vi "glueAlignPinInsert_stereo.vi"() -> ()   [LabVIEW 2015]
uses:
  GlobalPath.vi
  GlobalData.vi
  GlobalVi.vi
panel:
  in  "ptfe 42":bool caption="Manually push down the two pins of the vertical positioning tool to insert them in the holes of the plates"
  in  "ptfe 41":bool caption="Manually push down the two pins of the vertical positioning tool to insert them in the holes of the plates"
  out "PanelName":string
  in  "ptfe 33":bool caption="Remove the electroerosion pin"
  in  "ptfe 39":bool caption="Insert the electroerosition pin in the slotted insert"
  in  "ptfe 31":bool caption="Check the planarity of the tool with the gauge machine"
  in  "ptfe 30":bool caption="Tighten the three screws to block the vertical positioning tool in place"
  in  "ptfe 29":bool caption="Check the planarity of the tool with the gauge machine"
  in  "ptfe 28":bool caption="Tighten the three screws to block the vertical positioning tool in place"
  in  "ptfe 27":bool caption="Position the alignment pin in the panel hole"
  in  "ptfe 26":bool caption="Position the panel on the table"
  in  "ptfe 25":bool caption="Move the panel away from the table"
  in  "ptfe 24":bool caption="Lift the panel from the table"
  in  "ptfe 23":bool caption="Switch on the vacuum on the machine"
  in  "ptfe 22":bool caption="Lower the machine on the panel"
  in  "ptfe 21":bool caption="Move the rotating machine on top of the panel"
  in  "Done ?":bool
  in  "ptfe 20":bool caption="Wait 24h for the glue to cure"
  in  "ptfe 19":bool caption="Position the reinforcing washers on the emerging part of the alignment pins and insert"
  in  "ptfe 18":bool caption="Deposit the glue on the emerging part of the alignment pins and insert using a thin needle"
  in  "ptfe 17":bool caption="Rotate the panel so that it's back side is up"
  in  "ptfe 16":bool caption="Switch off the vacuum"
  in  "ptfe 15":bool caption="Remove the three vertical positioning tools, blocking plates and positioning pins"
  in  "ptfe 14":bool caption="Wait 24h for the glue to cure"
  in  "ptfe 13":bool caption="Place and screw the blocking plate to the vertical positioning tool to keep the pin orthogonality during the curing of the glue"
  in  "ptfe 12":bool caption="Position the vertical positioning tool on the reference plate with its positioning pins"
  in  "ptfe 11":bool caption="Deposit the glue on the stainless steel slotted insert grooves"
  in  "ptfe 9":bool caption="Position the insert in the dedicated hole on the panel"
  in  "ptfe 8":bool caption="Repeat these steps in order to glue the second alignment pin on the other side of the panel"
  in  "ptfe 7":bool caption="Place and screw the blocking plate to the vertical positioning tool to keep the pin orthogonality during the curing of the glue"
  in  "ptfe 5":bool caption="Position the vertical positioning tool on the reference plate with its positioning pins"
  in  "ptfe 4":bool caption="Deposit the glue on the precise alignment pin grooves"
  in  "ptfe 2":bool caption="Check that the vacuum is on"
  # "Gluing of Alignment Pin/Insert"
  # "STEREO PANEL \nINSTRUCTIONS"
  # "GLUING OF THE TWO PINS"
  # "GLUING OF THE HARDENED STEEL INSERT"
  # "Add info on Enumeration"
  # "COMMON PROCEDURE"
  # "GLUE CURING OF THE TWO PINS AND INSERT"
  # "GLUING OF REINFORCING WASHER ON PANEL BACK SIDE"
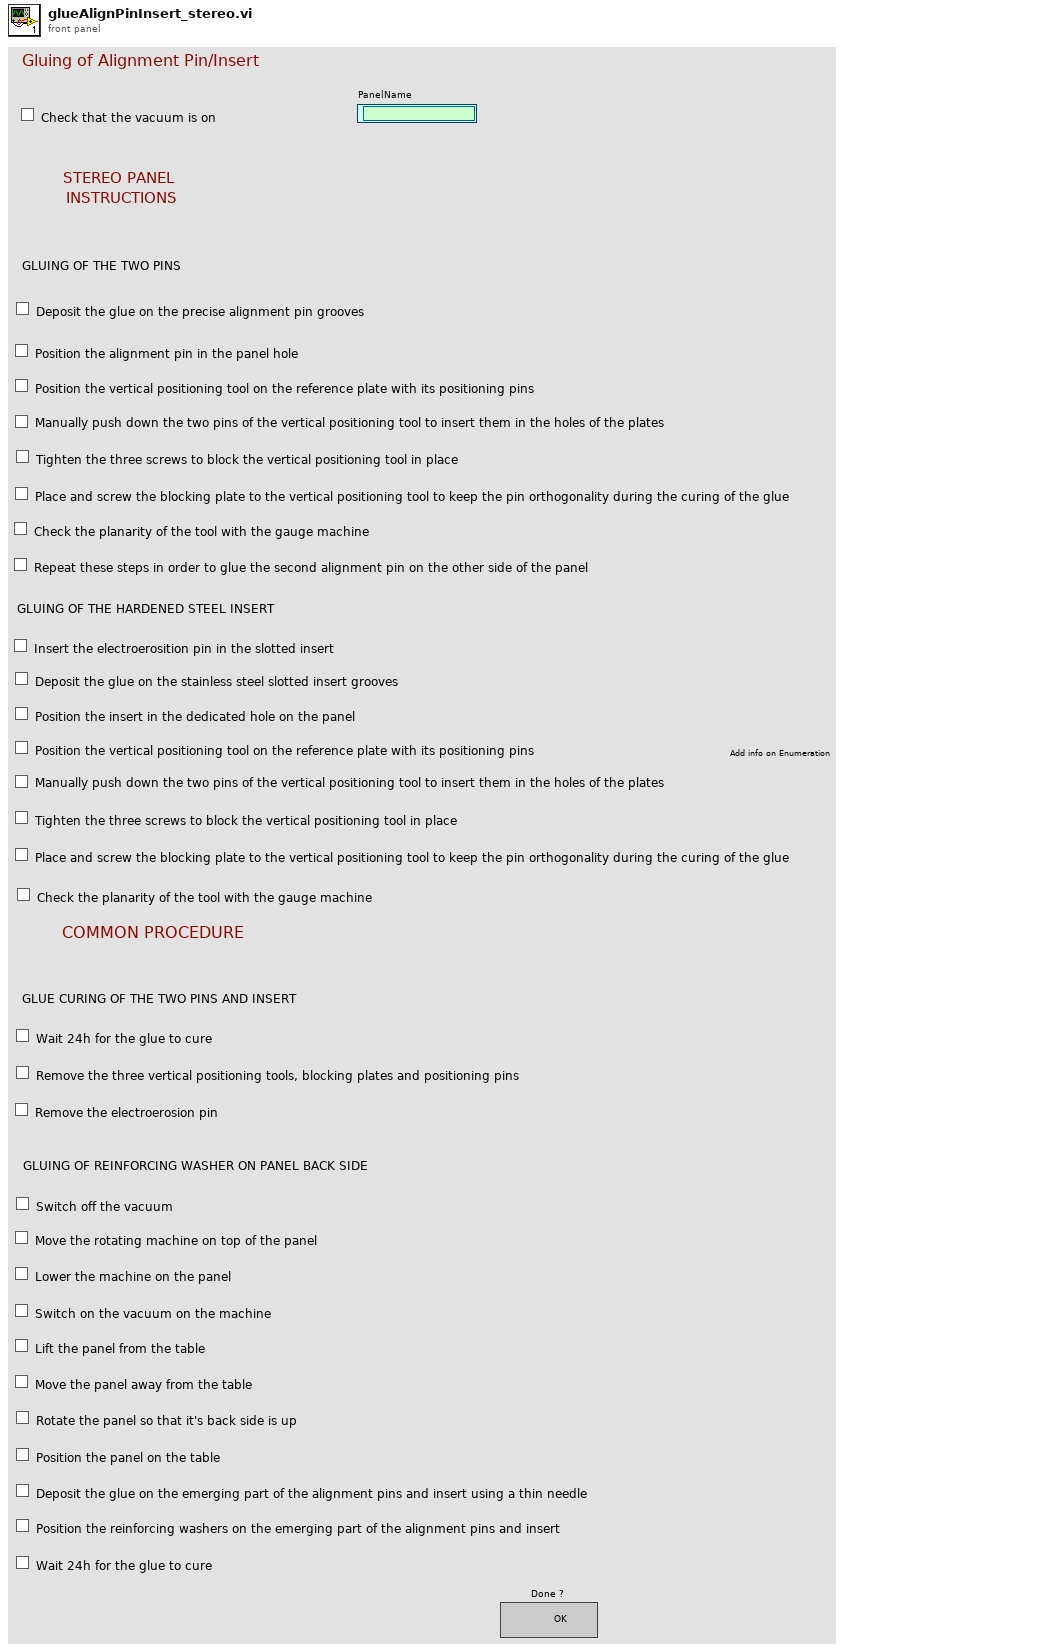
[diagram p1: front panel]
types:
  T1 = enum16{"open", "replace", "create", "open or create", "replace or create", "replace or create with confirmation"}
  T2 = enum32{"Bad", "Idle", "Run top level", "Running"}
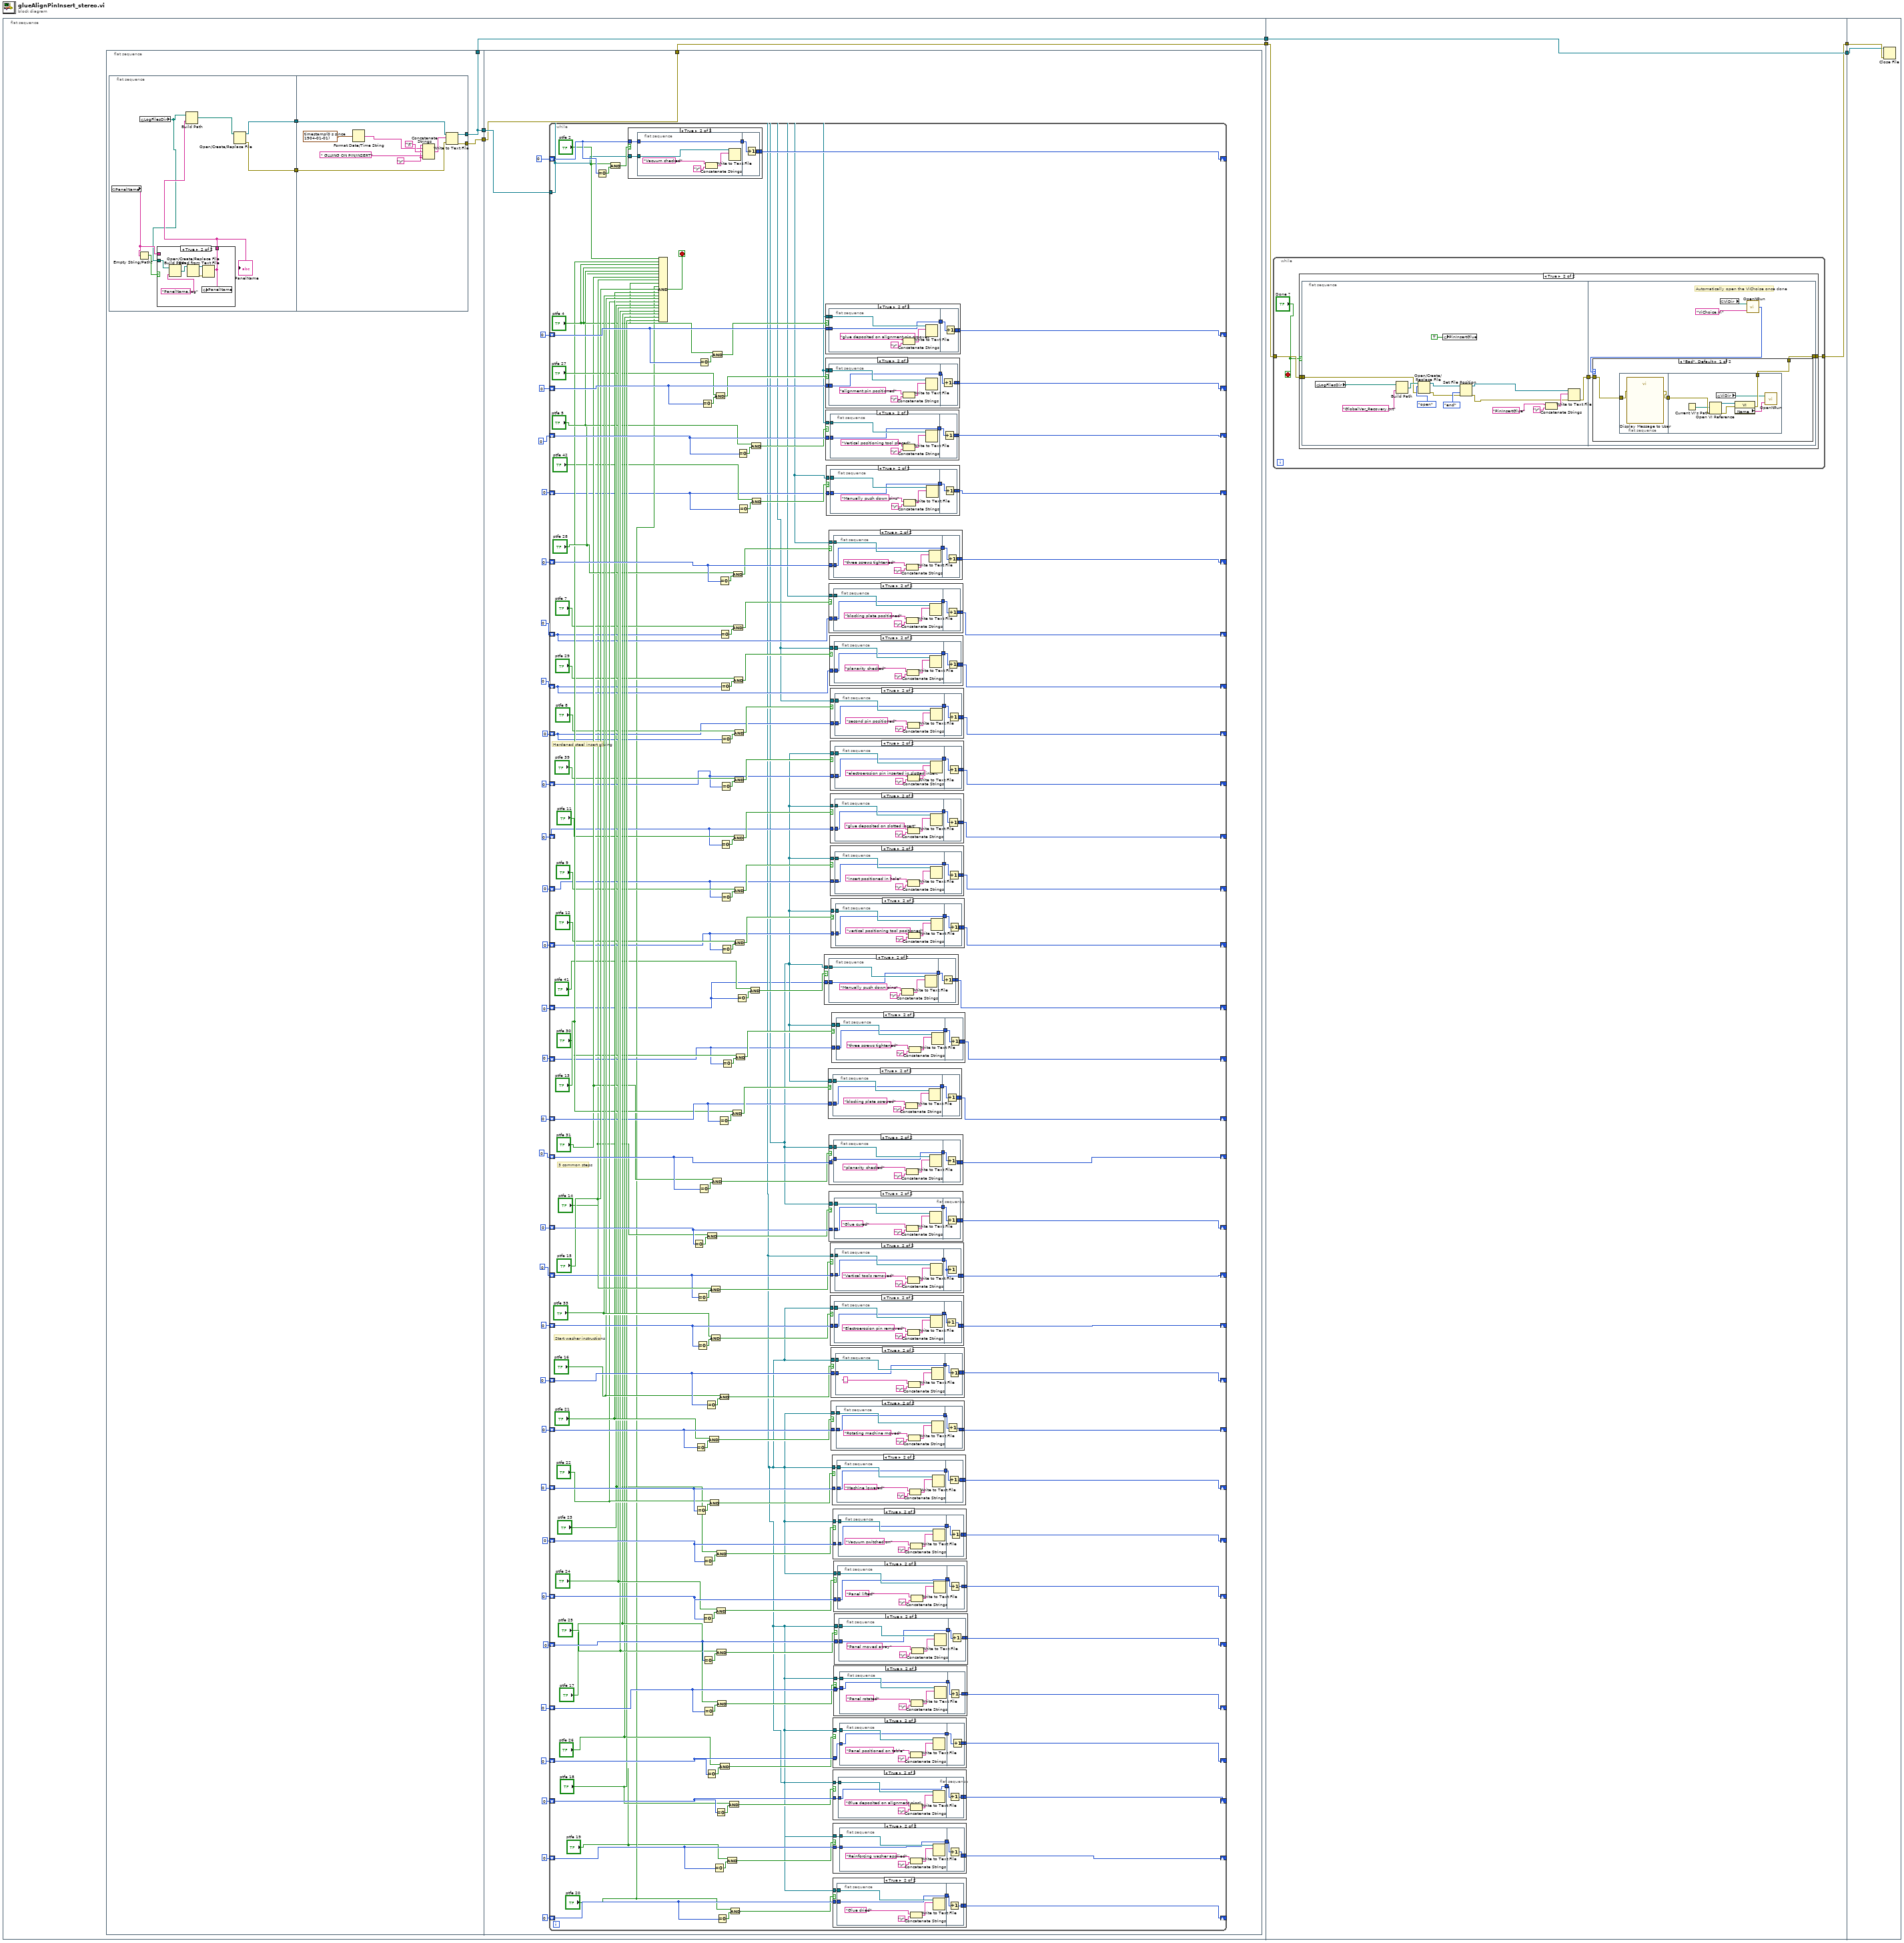
[diagram p0: block diagram]
diagram:
  n1 = flat-sequence {
    tunnel: [w5] -> w3
    tunnel: [w7] -> w2
    tunnel: [w598] -> w4
    tunnel: w3 -> [w599]
    tunnel: w2 -> [w600]
    tunnel: [w600] -> w1
    tunnel: w4 -> [w644]
    tunnel: w1 -> [w643]
    frame #0 {
      n2 = flat-sequence {
        tunnel: [w11] -> w8
        tunnel: [w11] -> w7
        tunnel: [w9] -> w6
        tunnel: w8 -> [w69]
        tunnel: w6 -> [w68]
        tunnel: [w68] -> w5
        frame #0 {
          n3 = flat-sequence {
            tunnel: [w18] -> w12
            tunnel: [w17] -> w10
            tunnel: w12 -> [w31]
            tunnel: [w30] -> w11
            tunnel: [w29] -> w9
            tunnel: w10 -> [w28]
            frame #0 {
              n4 = global read "GlobalData.vi" "PanelName"() -> (w16:string)
              n5 = Empty String/Path?(string/path=w16) -> (empty?=w15:bool)
              n6 = global read "GlobalPath.vi" "LogFilesDir"() -> (w13:path)
              n7 = case shown="True" w15 {
                tunnel: w13 -> [_ w26]
                tunnel: [w20 w21] -> w14
                tunnel: w16 -> [w20 _]
                frame False {
                }
                frame True {
                  n8 = Build Path(base path=w26, name or relative path="PanelName.log") -> (appended path=w25:path)
                  n9 = Open/Create/Replace File(file path (use dialog)=w25) -> (refnum out=w22:refnum<file>, error out=w23:errorcluster)  [unwired: 5 in, 1 out]
                  n10 = Read from Text File(file (use dialog)=w22, error in=w23) -> (text=w21:string)  [unwired: 2 in, 3 out]
                  n11 = global write "GlobalData.vi" "PanelName"(w21) -> ()
                }
              }
              "PanelName" <- w14
              n12 = Build Path(base path=w13, name or relative path=w14) -> (appended path=w19:path)
              n13 = Open/Create/Replace File(file path (use dialog)=w19) -> (refnum out=w18:refnum<file>, error out=w17:errorcluster)  [unwired: 5 in, 1 out]
            }
            frame #1 {
              w27 = "\r"
              n14 = Format Date/Time String(seconds (now)=timestamp(0 s since 1904-01-01)) -> (date/time string=w34:string)  [unwired: 2 in]
              n15 = Concatenate Strings(w27, w34, "\t", " GLUING ON PIN/INSERT", w27) -> (w32:string)
              n16 = Write to Text File(file (use dialog)=w31, text=w32, error in=w28) -> (refnum out=w30:refnum<file>, error out=w29:errorcluster)  [unwired: 1 in, 1 out]
            }
          }
        }
        frame #1 {
          n17 = while {
            tunnel: w69 -> [w73]
            shift-right: [w225] -> _
            shift-left: 0 -> [w204]
            shift-right: [w224] -> _
            shift-left: 0 -> [w196]
            shift-right: [w223] -> _
            shift-left: 0 -> [w195]
            shift-right: [w222] -> _
            shift-left: 0 -> [w194]
            shift-right: [w221] -> _
            shift-left: 0 -> [w190]
            shift-right: [w220] -> _
            shift-left: 0 -> [w188]
            shift-right: [w219] -> _
            shift-left: 0 -> [w183]
            shift-right: [w218] -> _
            shift-left: 0 -> [w180]
            shift-right: [w217] -> _
            shift-left: 0 -> [w178]
            shift-right: [w216] -> _
            shift-left: 0 -> [w167]
            shift-right: [w215] -> _
            shift-left: 0 -> [w166]
            shift-right: [w214] -> _
            shift-left: 0 -> [w165]
            shift-right: [w213] -> _
            shift-left: 0 -> [w164]
            shift-right: [w212] -> _
            shift-left: 0 -> [w163]
            shift-right: [w211] -> _
            shift-left: 0 -> [w162]
            shift-right: [w210] -> _
            shift-left: 0 -> [w161]
            shift-right: [w209] -> _
            shift-left: 0 -> [w160]
            shift-right: [w208] -> _
            shift-left: 0 -> [w159]
            shift-right: [w207] -> _
            shift-left: 0 -> [w139]
            shift-right: [w206] -> _
            shift-left: 0 -> [w138]
            shift-right: [w132] -> _
            shift-left: 0 -> [w133]
            shift-right: [w93] -> _
            shift-left: 0 -> [w101]
            shift-right: [w86] -> _
            shift-left: 0 -> [w100]
            shift-right: [w87] -> _
            shift-left: 0 -> [w99]
            shift-right: [w88] -> _
            shift-left: 0 -> [w98]
            shift-right: [w89] -> _
            shift-left: 0 -> [w97]
            shift-right: [w90] -> _
            shift-left: 0 -> [w96]
            shift-right: [w91] -> _
            shift-left: 0 -> [w95]
            shift-right: [w92] -> _
            shift-left: 0 -> [w94]
            shift-right: [w76] -> _
            shift-left: 0 -> [w77]
            shift-right: [w70] -> _
            shift-left: 0 -> [w71]
            stop <- w226 stop-if-true
            # "Hardened steel insert gluing"
            # "3 common steps"
            # "Start washer instructions"
            n18 = Equal To 0?(x=w204) -> (x = 0?=w205:bool)
            n19 = And(x="ptfe 2", y=w205) -> (x .and. y?=w202:bool)
            n20 = case shown="True" w202 {
              tunnel: w73 -> [_ w590]
              tunnel: w204 -> [w586 w589]
              tunnel: [w586 w587] -> w225
              frame False {
              }
              frame True {
                n21 = flat-sequence {
                  tunnel: w590 -> [w592]
                  tunnel: w589 -> [w591]
                  tunnel: [w591] -> w588
                  tunnel: w588 -> [w597]
                  tunnel: [w596] -> w587
                  frame #0 {
                    n22 = Concatenate Strings("Vacuum checked", "\r") -> (w595:string)
                    n23 = Write to Text File(file (use dialog)=w592, text=w595) -> ()  [unwired: 2 in, 3 out]
                  }
                  frame #1 {
                    n24 = Increment(x=w597) -> (x+1=w596:i32)
                  }
                }
              }
            }
            n25 = Compound Arithmetic op=AND("ptfe 2", "ptfe 13", "ptfe 4", "ptfe 4", "ptfe 5", "ptfe 28", "ptfe 31", "ptfe 14", "ptfe 19", "ptfe 20", "ptfe 15", "ptfe 21", "ptfe 33", "ptfe 16", "ptfe 22", "ptfe 23", "ptfe 24", "ptfe 25", "ptfe 17", "ptfe 26", "ptfe 18") -> (w226:bool)
            n26 = Equal To 0?(x=w183) -> (x = 0?=w186:bool)
            n27 = Equal To 0?(x=w166) -> (x = 0?=w175:bool)
            n28 = Equal To 0?(x=w165) -> (x = 0?=w174:bool)
            n29 = Equal To 0?(x=w180) -> (x = 0?=w185:bool)
            n30 = Equal To 0?(x=w178) -> (x = 0?=w184:bool)
            n31 = Equal To 0?(x=w188) -> (x = 0?=w197:bool)
            n32 = Equal To 0?(x=w196) -> (x = 0?=w201:bool)
            n33 = Equal To 0?(x=w195) -> (x = 0?=w200:bool)
            n34 = Equal To 0?(x=w163) -> (x = 0?=w172:bool)
            n35 = Equal To 0?(x=w164) -> (x = 0?=w173:bool)
            n36 = Equal To 0?(x=w162) -> (x = 0?=w171:bool)
            n37 = Equal To 0?(x=w161) -> (x = 0?=w170:bool)
            n38 = Equal To 0?(x=w167) -> (x = 0?=w176:bool)
            n39 = Equal To 0?(x=w160) -> (x = 0?=w169:bool)
            n40 = And(x="ptfe 14", y=w186) -> (x .and. y?=w182:bool)
            n41 = And(x="ptfe 21", y=w175) -> (x .and. y?=w154:bool)
            n42 = And(x="ptfe 22", y=w174) -> (x .and. y?=w152:bool)
            n43 = And(x="ptfe 15", y=w185) -> (x .and. y?=w179:bool)
            n44 = And(x="ptfe 33", y=w184) -> (x .and. y?=w177:bool)
            n45 = And(x="ptfe 31", y=w197) -> (x .and. y?=w187:bool)
            n46 = And(x="ptfe 4", y=w201) -> (x .and. y?=w193:bool)
            n47 = Equal To 0?(x=w139) -> (x = 0?=w141:bool)
            n48 = And(x="ptfe 27", y=w200) -> (x .and. y?=w192:bool)
            n49 = And(x="ptfe 24", y=w172) -> (x .and. y?=w150:bool)
            n50 = Equal To 0?(x=w159) -> (x = 0?=w168:bool)
            n51 = And(x="ptfe 23", y=w173) -> (x .and. y?=w85:bool)
            n52 = And(x="ptfe 25", y=w171) -> (x .and. y?=w148:bool)
            n53 = And(x="ptfe 17", y=w170) -> (x .and. y?=w146:bool)
            n54 = Equal To 0?(x=w138) -> (x = 0?=w140:bool)
            n55 = Equal To 0?(x=w133) -> (x = 0?=w135:bool)
            n56 = Equal To 0?(x=w190) -> (x = 0?=w198:bool)
            n57 = And(x="ptfe 16", y=w176) -> (x .and. y?=w156:bool)
            n58 = Equal To 0?(x=w100) -> (x = 0?=w125:bool)
            n59 = And(x="ptfe 26", y=w169) -> (x .and. y?=w144:bool)
            n60 = Equal To 0?(x=w99) -> (x = 0?=w123:bool)
            n61 = Equal To 0?(x=w96) -> (x = 0?=w117:bool)
            n62 = Equal To 0?(x=w98) -> (x = 0?=w121:bool)
            n63 = Equal To 0?(x=w97) -> (x = 0?=w119:bool)
            n64 = Equal To 0?(x=w95) -> (x = 0?=w115:bool)
            n65 = Equal To 0?(x=w94) -> (x = 0?=w113:bool)
            n66 = Equal To 0?(x=w101) -> (x = 0?=w111:bool)
            n67 = And(x="ptfe 19", y=w141) -> (x .and. y?=w137:bool)
            n68 = And(x="ptfe 18", y=w168) -> (x .and. y?=w142:bool)
            n69 = And(x="ptfe 20", y=w140) -> (x .and. y?=w136:bool)
            n70 = And(x="ptfe 13", y=w135) -> (x .and. y?=w134:bool)
            n71 = And(x="ptfe 28", y=w198) -> (x .and. y?=w189:bool)
            n72 = And(x="ptfe 7", y=w125) -> (x .and. y?=w124:bool)
            n73 = And(x="ptfe 29", y=w123) -> (x .and. y?=w122:bool)
            n74 = And(x="ptfe 11", y=w117) -> (x .and. y?=w116:bool)
            n75 = And(x="ptfe 8", y=w121) -> (x .and. y?=w120:bool)
            n76 = And(x="ptfe 39", y=w119) -> (x .and. y?=w118:bool)
            n77 = And(x="ptfe 9", y=w115) -> (x .and. y?=w114:bool)
            n78 = And(x="ptfe 12", y=w113) -> (x .and. y?=w112:bool)
            n79 = And(x="ptfe 30", y=w111) -> (x .and. y?=w110:bool)
            n80 = Equal To 0?(x=w71) -> (x = 0?=w75:bool)
            n81 = Equal To 0?(x=w194) -> (x = 0?=w199:bool)
            n82 = Equal To 0?(x=w77) -> (x = 0?=w80:bool)
            n83 = And(x="ptfe 41", y=w75) -> (x .and. y?=w74:bool)
            n84 = And(x="ptfe 5", y=w199) -> (x .and. y?=w191:bool)
            n85 = And(x="ptfe 42", y=w80) -> (x .and. y?=w79:bool)
            n86 = case shown="True" w74 {
              tunnel: w73 -> [_ w231]
              tunnel: w71 -> [w227 w229]
              tunnel: [w227 w228] -> w70
              frame False {
              }
              frame True {
                n87 = flat-sequence {
                  tunnel: w231 -> [w233]
                  tunnel: [w232] -> w230
                  tunnel: w229 -> [w232]
                  tunnel: w230 -> [w238]
                  tunnel: [w237] -> w228
                  frame #0 {
                    n88 = Concatenate Strings("Manually push down pins", "\r") -> (w236:string)
                    n89 = Write to Text File(file (use dialog)=w233, text=w236) -> ()  [unwired: 2 in, 3 out]
                  }
                  frame #1 {
                    n90 = Increment(x=w238) -> (x+1=w237:i32)
                  }
                }
              }
            }
            n91 = case shown="True" w192 {
              tunnel: w73 -> [_ w566]
              tunnel: w195 -> [w562 w564]
              tunnel: [w562 w563] -> w223
              frame False {
              }
              frame True {
                n92 = flat-sequence {
                  tunnel: w566 -> [w568]
                  tunnel: [w567] -> w565
                  tunnel: w564 -> [w567]
                  tunnel: w565 -> [w573]
                  tunnel: [w572] -> w563
                  frame #0 {
                    n93 = Concatenate Strings("alignment pin positioned", "\r") -> (w571:string)
                    n94 = Write to Text File(file (use dialog)=w568, text=w571) -> ()  [unwired: 2 in, 3 out]
                  }
                  frame #1 {
                    n95 = Increment(x=w573) -> (x+1=w572:i32)
                  }
                }
              }
            }
            n96 = case shown="True" w193 {
              tunnel: w73 -> [_ w578]
              tunnel: w196 -> [w574 w577]
              tunnel: [w574 w575] -> w224
              frame False {
              }
              frame True {
                n97 = flat-sequence {
                  tunnel: w578 -> [w580]
                  tunnel: w577 -> [w579]
                  tunnel: [w579] -> w576
                  tunnel: w576 -> [w585]
                  tunnel: [w584] -> w575
                  frame #0 {
                    n98 = Concatenate Strings("glue deposited on alignment pin grooves", "\r") -> (w583:string)
                    n99 = Write to Text File(file (use dialog)=w580, text=w583) -> ()  [unwired: 2 in, 3 out]
                  }
                  frame #1 {
                    n100 = Increment(x=w585) -> (x+1=w584:i32)
                  }
                }
              }
            }
            n101 = case shown="True" w191 {
              tunnel: w73 -> [_ w554]
              tunnel: w194 -> [w550 w552]
              tunnel: [w550 w551] -> w222
              frame False {
              }
              frame True {
                n102 = flat-sequence {
                  tunnel: w554 -> [w556]
                  tunnel: [w555] -> w553
                  tunnel: w552 -> [w555]
                  tunnel: w553 -> [w561]
                  tunnel: [w560] -> w551
                  frame #0 {
                    n103 = Concatenate Strings("Vertical positioning tool placed", "\r") -> (w559:string)
                    n104 = Write to Text File(file (use dialog)=w556, text=w559) -> ()  [unwired: 2 in, 3 out]
                  }
                  frame #1 {
                    n105 = Increment(x=w561) -> (x+1=w560:i32)
                  }
                }
              }
            }
            n106 = case shown="True" w79 {
              tunnel: w73 -> [_ w243]
              tunnel: w77 -> [w239 w241]
              tunnel: [w239 w240] -> w76
              frame False {
              }
              frame True {
                n107 = flat-sequence {
                  tunnel: w243 -> [w245]
                  tunnel: [w244] -> w242
                  tunnel: w241 -> [w244]
                  tunnel: w242 -> [w250]
                  tunnel: [w249] -> w240
                  frame #0 {
                    n108 = Concatenate Strings("Manually push down pins", "\r") -> (w248:string)
                    n109 = Write to Text File(file (use dialog)=w245, text=w248) -> ()  [unwired: 2 in, 3 out]
                  }
                  frame #1 {
                    n110 = Increment(x=w250) -> (x+1=w249:i32)
                  }
                }
              }
            }
            n111 = case shown="True" w134 {
              tunnel: w73 -> [_ w351]
              tunnel: w133 -> [w347 w349]
              tunnel: [w347 w348] -> w132
              frame False {
              }
              frame True {
                n112 = flat-sequence {
                  tunnel: w351 -> [w353]
                  tunnel: [w352] -> w350
                  tunnel: w349 -> [w352]
                  tunnel: w350 -> [w358]
                  tunnel: [w357] -> w348
                  frame #0 {
                    n113 = Concatenate Strings("blocking plate screwed", "\r") -> (w356:string)
                    n114 = Write to Text File(file (use dialog)=w353, text=w356) -> ()  [unwired: 2 in, 3 out]
                  }
                  frame #1 {
                    n115 = Increment(x=w358) -> (x+1=w357:i32)
                  }
                }
              }
            }
            n116 = case shown="True" w189 {
              tunnel: w73 -> [_ w530]
              tunnel: w190 -> [w526 w528]
              tunnel: [w526 w527] -> w221
              frame False {
              }
              frame True {
                n117 = flat-sequence {
                  tunnel: w530 -> [w532]
                  tunnel: [w531] -> w529
                  tunnel: w528 -> [w531]
                  tunnel: w529 -> [w537]
                  tunnel: [w536] -> w527
                  frame #0 {
                    n118 = Concatenate Strings("three screws tightened", "\r") -> (w535:string)
                    n119 = Write to Text File(file (use dialog)=w532, text=w535) -> ()  [unwired: 2 in, 3 out]
                  }
                  frame #1 {
                    n120 = Increment(x=w537) -> (x+1=w536:i32)
                  }
                }
              }
            }
            n121 = case shown="True" w124 {
              tunnel: w73 -> [_ w339]
              tunnel: w100 -> [w335 w337]
              tunnel: [w335 w336] -> w86
              frame False {
              }
              frame True {
                n122 = flat-sequence {
                  tunnel: w339 -> [w341]
                  tunnel: [w340] -> w338
                  tunnel: w337 -> [w340]
                  tunnel: w338 -> [w346]
                  tunnel: [w345] -> w336
                  frame #0 {
                    n123 = Concatenate Strings("blocking plate positioned", "\r") -> (w344:string)
                    n124 = Write to Text File(file (use dialog)=w341, text=w344) -> ()  [unwired: 2 in, 3 out]
                  }
                  frame #1 {
                    n125 = Increment(x=w346) -> (x+1=w345:i32)
                  }
                }
              }
            }
            n126 = case shown="True" w187 {
              tunnel: w73 -> [_ w542]
              tunnel: w188 -> [w538 w541]
              tunnel: [w538 w539] -> w220
              frame False {
              }
              frame True {
                n127 = flat-sequence {
                  tunnel: w542 -> [w544]
                  tunnel: w541 -> [w543]
                  tunnel: [w543] -> w540
                  tunnel: w540 -> [w549]
                  tunnel: [w548] -> w539
                  frame #0 {
                    n128 = Concatenate Strings("planarity checked", "\r") -> (w547:string)
                    n129 = Write to Text File(file (use dialog)=w544, text=w547) -> ()  [unwired: 2 in, 3 out]
                  }
                  frame #1 {
                    n130 = Increment(x=w549) -> (x+1=w548:i32)
                  }
                }
              }
            }
            n131 = case shown="True" w182 {
              tunnel: w73 -> [_ w518]
              tunnel: w183 -> [w514 w516]
              tunnel: [w514 w515] -> w219
              frame False {
              }
              frame True {
                n132 = flat-sequence {
                  tunnel: w518 -> [w520]
                  tunnel: [w519] -> w517
                  tunnel: w516 -> [w519]
                  tunnel: w517 -> [w525]
                  tunnel: [w524] -> w515
                  frame #0 {
                    n133 = Concatenate Strings("Glue cured", "\r") -> (w523:string)
                    n134 = Write to Text File(file (use dialog)=w520, text=w523) -> ()  [unwired: 2 in, 3 out]
                  }
                  frame #1 {
                    n135 = Increment(x=w525) -> (x+1=w524:i32)
                  }
                }
              }
            }
            n136 = case shown="True" w122 {
              tunnel: w73 -> [_ w327]
              tunnel: w99 -> [w323 w325]
              tunnel: [w323 w324] -> w87
              frame False {
              }
              frame True {
                n137 = flat-sequence {
                  tunnel: w327 -> [w329]
                  tunnel: [w328] -> w326
                  tunnel: w325 -> [w328]
                  tunnel: w326 -> [w334]
                  tunnel: [w333] -> w324
                  frame #0 {
                    n138 = Concatenate Strings("planarity checked", "\r") -> (w332:string)
                    n139 = Write to Text File(file (use dialog)=w329, text=w332) -> ()  [unwired: 2 in, 3 out]
                  }
                  frame #1 {
                    n140 = Increment(x=w334) -> (x+1=w333:i32)
                  }
                }
              }
            }
            n141 = case shown="True" w116 {
              tunnel: w73 -> [_ w291]
              tunnel: w96 -> [w287 w289]
              tunnel: [w287 w288] -> w90
              frame False {
              }
              frame True {
                n142 = flat-sequence {
                  tunnel: w291 -> [w293]
                  tunnel: [w292] -> w290
                  tunnel: w289 -> [w292]
                  tunnel: w290 -> [w298]
                  tunnel: [w297] -> w288
                  frame #0 {
                    n143 = Concatenate Strings("glue deposited on slotted insert", "\r") -> (w296:string)
                    n144 = Write to Text File(file (use dialog)=w293, text=w296) -> ()  [unwired: 2 in, 3 out]
                  }
                  frame #1 {
                    n145 = Increment(x=w298) -> (x+1=w297:i32)
                  }
                }
              }
            }
            n146 = case shown="True" w179 {
              tunnel: w73 -> [_ w507]
              tunnel: w180 -> [w503 w505]
              tunnel: [w503 w504] -> w218
              frame False {
              }
              frame True {
                n147 = flat-sequence {
                  tunnel: w507 -> [w509]
                  tunnel: [w508] -> w506
                  tunnel: w505 -> [w508]
                  tunnel: w506 -> [w513]
                  tunnel: [w513] -> w504
                  frame #0 {
                    n148 = Concatenate Strings("Vertical tools removed", "\r") -> (w512:string)
                    n149 = Write to Text File(file (use dialog)=w509, text=w512) -> ()  [unwired: 2 in, 3 out]
                  }
                  frame #1 {
                    n150 = Increment(x=w513) -> ()  [unwired: 1 out]
                  }
                }
              }
            }
            n151 = case shown="True" w177 {
              tunnel: w73 -> [_ w495]
              tunnel: w178 -> [w491 w493]
              tunnel: [w491 w492] -> w217
              frame False {
              }
              frame True {
                n152 = flat-sequence {
                  tunnel: w495 -> [w497]
                  tunnel: [w496] -> w494
                  tunnel: w493 -> [w496]
                  tunnel: w494 -> [w502]
                  tunnel: [w501] -> w492
                  frame #0 {
                    n153 = Concatenate Strings("Electroerosion pin removed", "\r") -> (w500:string)
                    n154 = Write to Text File(file (use dialog)=w497, text=w500) -> ()  [unwired: 2 in, 3 out]
                  }
                  frame #1 {
                    n155 = Increment(x=w502) -> (x+1=w501:i32)
                  }
                }
              }
            }
            n156 = case shown="True" w120 {
              tunnel: w73 -> [_ w315]
              tunnel: w98 -> [w311 w313]
              tunnel: [w311 w312] -> w88
              frame False {
              }
              frame True {
                n157 = flat-sequence {
                  tunnel: w315 -> [w317]
                  tunnel: [w316] -> w314
                  tunnel: w313 -> [w316]
                  tunnel: w314 -> [w322]
                  tunnel: [w321] -> w312
                  frame #0 {
                    n158 = Concatenate Strings("second pin positioned", "\r") -> (w320:string)
                    n159 = Write to Text File(file (use dialog)=w317, text=w320) -> ()  [unwired: 2 in, 3 out]
                  }
                  frame #1 {
                    n160 = Increment(x=w322) -> (x+1=w321:i32)
                  }
                }
              }
            }
            n161 = case shown="True" w118 {
              tunnel: w73 -> [_ w303]
              tunnel: w97 -> [w299 w301]
              tunnel: [w299 w300] -> w89
              frame False {
              }
              frame True {
                n162 = flat-sequence {
                  tunnel: w303 -> [w305]
                  tunnel: [w304] -> w302
                  tunnel: w301 -> [w304]
                  tunnel: w302 -> [w310]
                  tunnel: [w309] -> w300
                  frame #0 {
                    n163 = Concatenate Strings("electroerosion pin inserted in slotted insert", "\r") -> (w308:string)
                    n164 = Write to Text File(file (use dialog)=w305, text=w308) -> ()  [unwired: 2 in, 3 out]
                  }
                  frame #1 {
                    n165 = Increment(x=w310) -> (x+1=w309:i32)
                  }
                }
              }
            }
            n166 = case shown="True" w114 {
              tunnel: w73 -> [_ w279]
              tunnel: w95 -> [w275 w277]
              tunnel: [w275 w276] -> w91
              frame False {
              }
              frame True {
                n167 = flat-sequence {
                  tunnel: w279 -> [w281]
                  tunnel: [w280] -> w278
                  tunnel: w277 -> [w280]
                  tunnel: w278 -> [w286]
                  tunnel: [w285] -> w276
                  frame #0 {
                    n168 = Concatenate Strings("insert positioned in hole", "\r") -> (w284:string)
                    n169 = Write to Text File(file (use dialog)=w281, text=w284) -> ()  [unwired: 2 in, 3 out]
                  }
                  frame #1 {
                    n170 = Increment(x=w286) -> (x+1=w285:i32)
                  }
                }
              }
            }
            n171 = case shown="True" w112 {
              tunnel: w73 -> [_ w267]
              tunnel: w94 -> [w263 w265]
              tunnel: [w263 w264] -> w92
              frame False {
              }
              frame True {
                n172 = flat-sequence {
                  tunnel: w267 -> [w269]
                  tunnel: [w268] -> w266
                  tunnel: w265 -> [w268]
                  tunnel: w266 -> [w274]
                  tunnel: [w273] -> w264
                  frame #0 {
                    n173 = Concatenate Strings("vertical positioning tool positioned", "\r") -> (w272:string)
                    n174 = Write to Text File(file (use dialog)=w269, text=w272) -> ()  [unwired: 2 in, 3 out]
                  }
                  frame #1 {
                    n175 = Increment(x=w274) -> (x+1=w273:i32)
                  }
                }
              }
            }
            n176 = case shown="True" w156 {
              tunnel: w73 -> [_ w483]
              tunnel: w167 -> [w479 w481]
              tunnel: [w479 w480] -> w216
              frame False {
              }
              frame True {
                n177 = flat-sequence {
                  tunnel: w483 -> [w485]
                  tunnel: [w484] -> w482
                  tunnel: w481 -> [w484]
                  tunnel: w482 -> [w490]
                  tunnel: [w489] -> w480
                  frame #0 {
                    n178 = Concatenate Strings("\u0000", "\r") -> (w488:string)
                    n179 = Write to Text File(file (use dialog)=w485, text=w488) -> ()  [unwired: 2 in, 3 out]
                  }
                  frame #1 {
                    n180 = Increment(x=w490) -> (x+1=w489:i32)
                  }
                }
              }
            }
            n181 = case shown="True" w154 {
              tunnel: w73 -> [_ w471]
              tunnel: w166 -> [w467 w469]
              tunnel: [w467 w468] -> w215
              frame False {
              }
              frame True {
                n182 = flat-sequence {
                  tunnel: w471 -> [w473]
                  tunnel: [w472] -> w470
                  tunnel: w469 -> [w472]
                  tunnel: w470 -> [w478]
                  tunnel: [w477] -> w468
                  frame #0 {
                    n183 = Concatenate Strings("Rotating machine moved", "\r") -> (w476:string)
                    n184 = Write to Text File(file (use dialog)=w473, text=w476) -> ()  [unwired: 2 in, 3 out]
                  }
                  frame #1 {
                    n185 = Increment(x=w478) -> (x+1=w477:i32)
                  }
                }
              }
            }
            n186 = case shown="True" w110 {
              tunnel: w73 -> [_ w255]
              tunnel: w101 -> [w251 w253]
              tunnel: [w251 w252] -> w93
              frame False {
              }
              frame True {
                n187 = flat-sequence {
                  tunnel: w255 -> [w257]
                  tunnel: [w256] -> w254
                  tunnel: w253 -> [w256]
                  tunnel: w254 -> [w262]
                  tunnel: [w261] -> w252
                  frame #0 {
                    n188 = Concatenate Strings("three screws tightened", "\r") -> (w260:string)
                    n189 = Write to Text File(file (use dialog)=w257, text=w260) -> ()  [unwired: 2 in, 3 out]
                  }
                  frame #1 {
                    n190 = Increment(x=w262) -> (x+1=w261:i32)
                  }
                }
              }
            }
            n191 = case shown="True" w152 {
              tunnel: w73 -> [_ w459]
              tunnel: w165 -> [w455 w457]
              tunnel: [w455 w456] -> w214
              frame False {
              }
              frame True {
                n192 = flat-sequence {
                  tunnel: w459 -> [w461]
                  tunnel: [w460] -> w458
                  tunnel: w457 -> [w460]
                  tunnel: w458 -> [w466]
                  tunnel: [w465] -> w456
                  frame #0 {
                    n193 = Concatenate Strings("Machine lowered", "\r") -> (w464:string)
                    n194 = Write to Text File(file (use dialog)=w461, text=w464) -> ()  [unwired: 2 in, 3 out]
                  }
                  frame #1 {
                    n195 = Increment(x=w466) -> (x+1=w465:i32)
                  }
                }
              }
            }
            n196 = case shown="True" w85 {
              tunnel: w73 -> [_ w447]
              tunnel: w164 -> [w443 w445]
              tunnel: [w443 w444] -> w213
              frame False {
              }
              frame True {
                n197 = flat-sequence {
                  tunnel: w447 -> [w449]
                  tunnel: [w448] -> w446
                  tunnel: w445 -> [w448]
                  tunnel: w446 -> [w454]
                  tunnel: [w453] -> w444
                  frame #0 {
                    n198 = Concatenate Strings("Vacuum switched on", "\r") -> (w452:string)
                    n199 = Write to Text File(file (use dialog)=w449, text=w452) -> ()  [unwired: 2 in, 3 out]
                  }
                  frame #1 {
                    n200 = Increment(x=w454) -> (x+1=w453:i32)
                  }
                }
              }
            }
            n201 = case shown="True" w142 {
              tunnel: w73 -> [_ w399]
              tunnel: w159 -> [w395 w397]
              tunnel: [w395 w396] -> w208
              frame False {
              }
              frame True {
                n202 = flat-sequence {
                  tunnel: w399 -> [w401]
                  tunnel: [w400] -> w398
                  tunnel: w397 -> [w400]
                  tunnel: w398 -> [w406]
                  tunnel: [w405] -> w396
                  frame #0 {
                    n203 = Concatenate Strings("Glue deposited on alignment pins", "\r") -> (w404:string)
                    n204 = Write to Text File(file (use dialog)=w401, text=w404) -> ()  [unwired: 2 in, 3 out]
                  }
                  frame #1 {
                    n205 = Increment(x=w406) -> (x+1=w405:i32)
                  }
                }
              }
            }
            n206 = case shown="True" w136 {
              tunnel: w73 -> [_ w375]
              tunnel: w138 -> [w371 w374]
              tunnel: [w371 w372] -> w206
              frame False {
              }
              frame True {
                n207 = flat-sequence {
                  tunnel: w375 -> [w377]
                  tunnel: w374 -> [w376]
                  tunnel: [w376] -> w373
                  tunnel: w373 -> [w382]
                  tunnel: [w381] -> w372
                  frame #0 {
                    n208 = Concatenate Strings("Glue dried", "\r") -> (w380:string)
                    n209 = Write to Text File(file (use dialog)=w377, text=w380) -> ()  [unwired: 2 in, 3 out]
                  }
                  frame #1 {
                    n210 = Increment(x=w382) -> (x+1=w381:i32)
                  }
                }
              }
            }
            n211 = case shown="True" w144 {
              tunnel: w73 -> [_ w411]
              tunnel: w160 -> [w407 w410]
              tunnel: [w407 w408] -> w209
              frame False {
              }
              frame True {
                n212 = flat-sequence {
                  tunnel: w411 -> [w413]
                  tunnel: w410 -> [w412]
                  tunnel: [w412] -> w409
                  tunnel: w409 -> [w418]
                  tunnel: [w417] -> w408
                  frame #0 {
                    n213 = Concatenate Strings("Panel positioned on table", "\r") -> (w416:string)
                    n214 = Write to Text File(file (use dialog)=w413, text=w416) -> ()  [unwired: 2 in, 3 out]
                  }
                  frame #1 {
                    n215 = Increment(x=w418) -> (x+1=w417:i32)
                  }
                }
              }
            }
            n216 = case shown="True" w137 {
              tunnel: w73 -> [_ w387]
              tunnel: w139 -> [w383 w385]
              tunnel: [w383 w384] -> w207
              frame False {
              }
              frame True {
                n217 = flat-sequence {
                  tunnel: w387 -> [w389]
                  tunnel: [w388] -> w386
                  tunnel: w385 -> [w388]
                  tunnel: w386 -> [w394]
                  tunnel: [w393] -> w384
                  frame #0 {
                    n218 = Concatenate Strings("Reinforcing washer applied", "\r") -> (w392:string)
                    n219 = Write to Text File(file (use dialog)=w389, text=w392) -> ()  [unwired: 2 in, 3 out]
                  }
                  frame #1 {
                    n220 = Increment(x=w394) -> (x+1=w393:i32)
                  }
                }
              }
            }
            n221 = case shown="True" w150 {
              tunnel: w73 -> [_ w435]
              tunnel: w163 -> [w431 w433]
              tunnel: [w431 w432] -> w212
              frame False {
              }
              frame True {
                n222 = flat-sequence {
                  tunnel: w435 -> [w437]
                  tunnel: [w436] -> w434
                  tunnel: w433 -> [w436]
                  tunnel: w434 -> [w442]
                  tunnel: [w441] -> w432
                  frame #0 {
                    n223 = Concatenate Strings("Panel lifted", "\r") -> (w440:string)
                    n224 = Write to Text File(file (use dialog)=w437, text=w440) -> ()  [unwired: 2 in, 3 out]
                  }
                  frame #1 {
                    n225 = Increment(x=w442) -> (x+1=w441:i32)
                  }
                }
              }
            }
            n226 = case shown="True" w146 {
              tunnel: w73 -> [_ w363]
              tunnel: w161 -> [w359 w362]
              tunnel: [w359 w360] -> w210
              frame False {
              }
              frame True {
                n227 = flat-sequence {
                  tunnel: w363 -> [w365]
                  tunnel: w362 -> [w364]
                  tunnel: [w364] -> w361
                  tunnel: w361 -> [w370]
                  tunnel: [w369] -> w360
                  frame #0 {
                    n228 = Concatenate Strings("Panel rotated", "\r") -> (w368:string)
                    n229 = Write to Text File(file (use dialog)=w365, text=w368) -> ()  [unwired: 2 in, 3 out]
                  }
                  frame #1 {
                    n230 = Increment(x=w370) -> (x+1=w369:i32)
                  }
                }
              }
            }
            n231 = case shown="True" w148 {
              tunnel: w73 -> [_ w423]
              tunnel: w162 -> [w419 w421]
              tunnel: [w419 w420] -> w211
              frame False {
              }
              frame True {
                n232 = flat-sequence {
                  tunnel: w423 -> [w425]
                  tunnel: [w424] -> w422
                  tunnel: w421 -> [w424]
                  tunnel: w422 -> [w430]
                  tunnel: [w429] -> w420
                  frame #0 {
                    n233 = Concatenate Strings("Panel moved away", "\r") -> (w428:string)
                    n234 = Write to Text File(file (use dialog)=w425, text=w428) -> ()  [unwired: 2 in, 3 out]
                  }
                  frame #1 {
                    n235 = Increment(x=w430) -> (x+1=w429:i32)
                  }
                }
              }
            }
          }
        }
      }
    }
    frame #1 {
      n236 = while {
        tunnel: [w603] -> w598
        tunnel: w599 -> [w602]
        stop <- "Done ?" stop-if-true
        n237 = case shown="True" "Done ?" {
          tunnel: [w604 w607] -> w603
          tunnel: w602 -> [w604 w606]
          frame False {
          }
          frame True {
            n238 = flat-sequence {
              tunnel: w606 -> [w611]
              tunnel: [w610] -> w605
              tunnel: [w624] -> w607
              tunnel: w605 -> [w623]
              frame #0 {
                n239 = global read "GlobalPath.vi" "LogFilesDir"() -> (w608:path)
                n240 = Build Path(base path=w608, name or relative path="GlobalVar_Recovery.txt") -> (appended path=w620:path)
                n241 = Open/Create/Replace File(file path (use dialog)=w620, error in=w611, operation (0:open)=T1."open") -> (refnum out=w616:refnum<file>, error out=w617:errorcluster)  [unwired: 3 in, 1 out]
                n242 = global write "GlobalVi.vi" "PinInsertGlue"(TRUE) -> ()
                n243 = Set File Position(refnum=w616, from (0:start)=enum16{"start", "end", "current"}."end", error in=w617) -> (refnum out=w613:refnum<file>, error out=w612:errorcluster)  [unwired: 1 in]
                n244 = Concatenate Strings("PinInsertGlue", "\r") -> (w615:string)
                n245 = Write to Text File(file (use dialog)=w613, text=w615, error in=w612) -> (error out=w610:errorcluster)  [unwired: 1 in, 2 out]
              }
              frame #1 {
                # "Automatically open the ViChoise once done"
                n246 = global read "GlobalPath.vi" "ViDir"() -> (w627:path)
                n247 = call "OpenNRun.vi"("VI name"="ViChoice.vi", "ViDirPath"=w627) -> ("Execution:State"=w626:T2)
                n248 = case shown="\"Bad\", Default" w626 {
                  tunnel: [w628 w640] -> w624
                  tunnel: w623 -> [w629 w640]
                  frame "Bad", Default {
                    n249 = flat-sequence {
                      tunnel: w629 -> [w632]
                      tunnel: [w631] -> w630
                      tunnel: [w636] -> w628
                      tunnel: w630 -> [w635]
                      frame #0 {
                        n250 = call "Display Message to User"("error in (no error)"=w632) -> ("error out"=w631:errorcluster)  [unwired: 9 in, 1 out]
                      }
                      frame #1 {
                        n251 = Current VI's Path() -> (path=w633:path)
                        n252 = Open VI Reference(vi path=w633, error in (no error)=w635) -> (vi reference=w639:refnum<vi>, error out=w638:errorcluster)  [unwired: 4 in]
                        n253 = global read "GlobalPath.vi" "ViDir"() -> (w634:path)
                        n254 = property class="VI"(reference=w639, error in=w638) -> (error out=w636:errorcluster, "Name"=w637:string)  [unwired: 1 out]
                        n255 = call "OpenNRun.vi"("VI name"=w637, "ViDirPath"=w634) -> ()  [unwired: 1 out]
                      }
                    }
                  }
                  frame "Idle" {
                    n256 = Current VI's Path() -> (path=w641:path)
                    n257 = Strip Path(path=w641) -> (name=w642:string)  [unwired: 1 out]
                    n258 = call <vilib>:"Close Panel.vi"("VI name"=w642) -> ()  [unwired: 10 in, 1 out]
                  }
                }
              }
            }
          }
        }
      }
    }
    frame #2 {
      n259 = Close File(refnum=w643, error in=w644) -> ()  [unwired: 2 out]
    }
  }
